vi "Is Winch PTO Engaged.vi"() -> (3 "Engaged?":bool)   [LabVIEW 2019]
doc: "This template is useful for immediate subsystem actions that do not need deadband filtering\n\nBe sure to right-click and select New from Template and save with a new command name."
uses:
  Implementation/Winch PTO State.vi
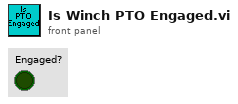
[diagram p1: front panel]
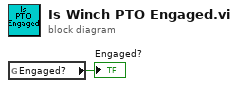
[diagram p0: block diagram]
diagram:
  n1 = global read "Winch PTO State.vi" "Engaged?"() -> (→"Engaged?":bool)
